vi "Concatenate Strings.vi"() -> ()   [LabVIEW 2016]
panel:
  out "String":string
  in  "String 2":string
  in  "String 1":string
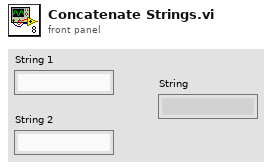
[diagram p1: front panel]
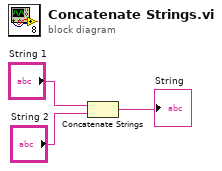
[diagram p0: block diagram]
diagram:
  n1 = Concatenate Strings("String 1", "String 2") -> (→"String":string)
